vi "Run.vi"(7 "Team Index":i32, 8 "Column":i32, 9 "Row":i32, 10 "View":i32[](array[numeric]) caption="View (Team Index, -1: empty)", 11 "Galaxy In":refnum<class "Galaxy.lvclass">) -> (0 "Replicated":refnum<class "Square.lvclass">, 1 "Direction":T1, 2 "Action":T2, 3 "Square Out":refnum<class "Square.lvclass">)   [LabVIEW 2020, in "Galaxy.lvclass"]
uses:
  Galaxy.lvclass
  C:/dev/IlluminatedG/sol-squarebattle/Square/Square.lvclass
  Square/Square.lvclass
  Type Defs/Action Enum.ctl
  Type Defs/Direction Enum.ctl
  SubVIs/Read-Only Globals.vi
  SubVIs/Globals (private).vi
  Common/Common.lvlib
  Type Defs/SB Type Defs.lvlib
panel:
  # "NW\nN\nNE\nE\nSE\nS\nSW\nW"
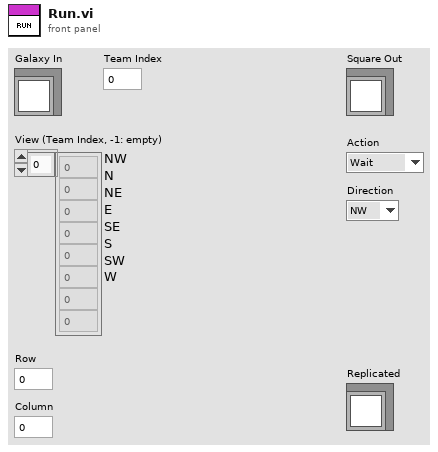
[diagram p1: front panel]
types:
  T1 = typedef "SB Type Defs.lvlib/Direction Enum.ctl" = enum16{"NW", "N", "NE", "E", "SE", "S", "SW", "W"}
  T2 = typedef "SB Type Defs.lvlib/Action Enum.ctl" = enum16{"Wait", "Move", "Attack", "Replicate"}
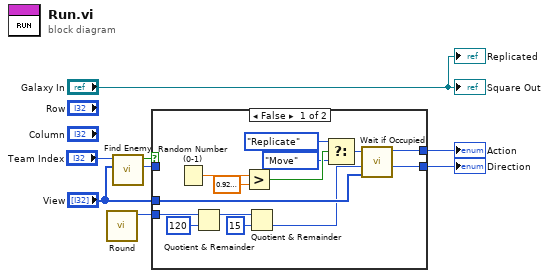
[diagram p0: block diagram]
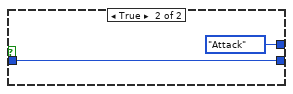
[diagram p2: hidden frame]
diagram:
  n1 = call "Round.vi"() -> ("Round"=w2:i32)  [unwired: 11 in]
  n2 = call "Find Enemy.vi"("View"="View", "Team Index"="Team Index") -> ("Direction"=w4:T1, "Found Enemy?"=w6:bool)  [unwired: 7 in, 1 out]
  n3 = case shown="False" w6 {
    tunnel: [w14 Action_Enum."Attack" ("Action")] -> w5
    tunnel: w4 -> [_ w23]
    tunnel: [w13 w23] -> w3
    tunnel: w2 -> [w17 _]
    tunnel: "View" -> [w12 _]
    frame False {
      n4 = Random Number (0-1)() -> (number: 0 to 1=w22:dbl)
      n5 = Quotient & Remainder(x=w17, y=120) -> (x-y*floor(x/y)=w10:i32)  [unwired: 1 out]
      n6 = Greater?(x=w22, y=0.9299999999999999) -> (0:w20:bool)
      n7 = Quotient & Remainder(x=w10, y=15) -> (floor(x/y)=w9:i32)  [unwired: 1 out]
      n8 = Select(t=Action_Enum."Replicate" ("Action"), s=w20, f=Action_Enum."Move" ("Action")) -> (s? t:f=w15:T2)
      n9 = call "Wait if Occupied.vi"("View"=w12, "Direction In"=w9, "Action In"=w15) -> ("Direction Out"=w13:T1, "Action Out"=w14:T2)  [unwired: 7 in]
    }
    frame True {
    }
  }
  "Action" <- w5
  "Direction" <- w3
  "Square Out" <- "Galaxy In"
  "Replicated" <- "Galaxy In"
